vi "Set_Sub_Collection.vi"(8 "error in (no error)":errorcluster caption="entrée d'erreur (pas d'erreur)", 11 "Firebase PCBA en entrée":refnum<class "Firebase AssembledProducts.lvclass">) -> (0 "error out":errorcluster caption="sortie d'erreur", 3 "Firebase PCBA en sortie":refnum<class "Firebase AssembledProducts.lvclass">)   [LabVIEW 2020, in "Library Instrument & Equipement.lvlib" / "Library FireBase.lvlib" / "Firebase AssembledProducts.lvclass"]
doc: "Create New document\nPlease initialise the following values\n - Name BDD\n - Document of test sequence\n - API Key"
uses:
  Firebase AssembledProducts.lvclass
  C:/Users/ngarcin/OneDrive - Altyor/Standard TB/Class/Firebase/Source/Firebase Driver/Firebase Driver.lvclass
  Firebase Altyor/Firebase Altyor.lvclass
  Firebase AssembledProducts.lvclass/Firebase AssembledProducts.ctl
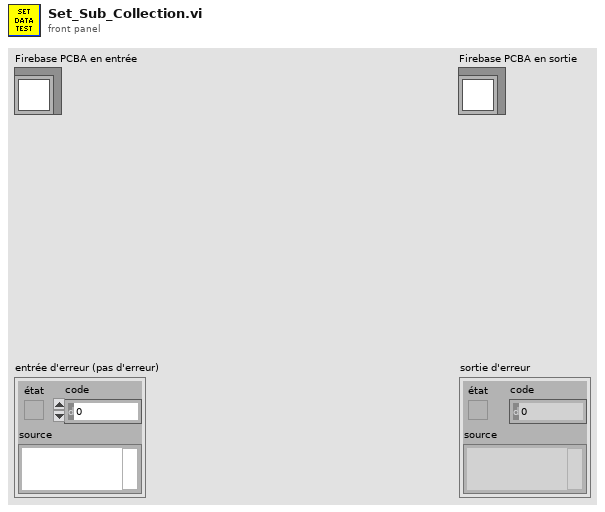
[diagram p1: front panel]
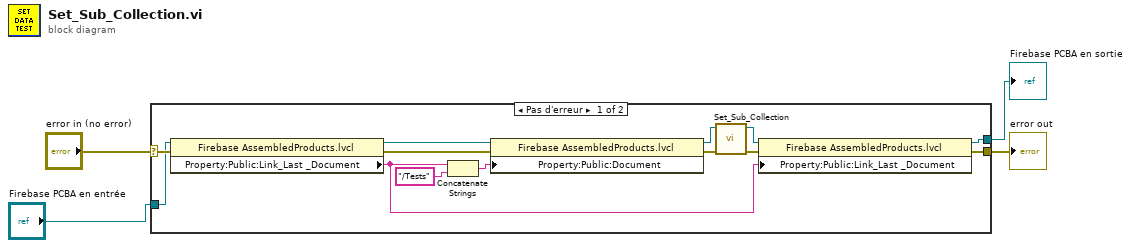
[diagram p0: block diagram]
diagram:
  n1 = case shown="Pas d'erreur" "error in (no error)" {
    selector: "error in (no error)" -> [w13 w19]
    tunnel: [w9 w19] -> w2
    tunnel: [w7 w18] -> w1
    tunnel: "Firebase PCBA en entrée" -> [w5 w18]
    frame No Error {
      n2 = property class="Firebase AssembledProducts.lvcl"(reference=w5, error in=w13) -> (reference out=w16:refnum<class "Firebase AssembledProducts.lvclass">, error out=w15:errorcluster, "Property:Public:Link_Last _Document"=w6:string)
      n3 = Concatenate Strings(w6, "/Tests" ("chaîne")) -> (w14:string)
      n4 = property class="Firebase AssembledProducts.lvcl"(reference=w16, error in=w15, "Property:Public:Document"=w14) -> (reference out=w12:refnum<class "Firebase AssembledProducts.lvclass">, error out=w11:errorcluster)
      n5 = call-parent "Set_Sub_Collection.vi"("error in (no error)"=w11, "Firebase PCBA en entrée"=w12) -> ("error out"=w10:errorcluster, "Firebase PCBA en sortie"=w8:refnum<class "Firebase AssembledProducts.lvclass">)  [unwired: 8 in]
      n6 = property class="Firebase AssembledProducts.lvcl"(reference=w8, error in=w10, "Property:Public:Link_Last _Document"=w6) -> (reference out=w7:refnum<class "Firebase AssembledProducts.lvclass">, error out=w9:errorcluster)
    }
    frame Error {
    }
  }
  "error out" <- w2
  "Firebase PCBA en sortie" <- w1
